vi "EnFlo_Seeder_Control.vi"(0 "Current Time (s)":dbl) -> ()   [LabVIEW 2014]
panel:
  in  "Minium Seeder power setting (Pmin)":dbl=27.0
  in  "Minimum Transducer Setting (Tmin)":dbl=6.0
  in  "Fluid Flowrate Factor":dbl=1.2 min=0.2 max=4.0 step=0.1 format="%.1g"
  in  "Sugar Strength":dbl=0.23
  out "Leak Detected or Emergency Stop":bool
  in  "Performing hand clean":bool
  out "Run Transducer":bool
  out "Sugar Pump":bool
  out "Low Flow":bool
  out "High Flow":bool
  out "Time Since Last Flush (min)":dbl
  out "Running Flush time":dbl
  out "Transducer setting":dbl
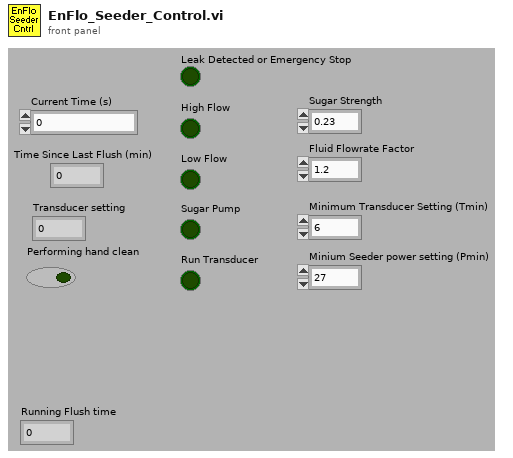
[diagram p1: front panel]
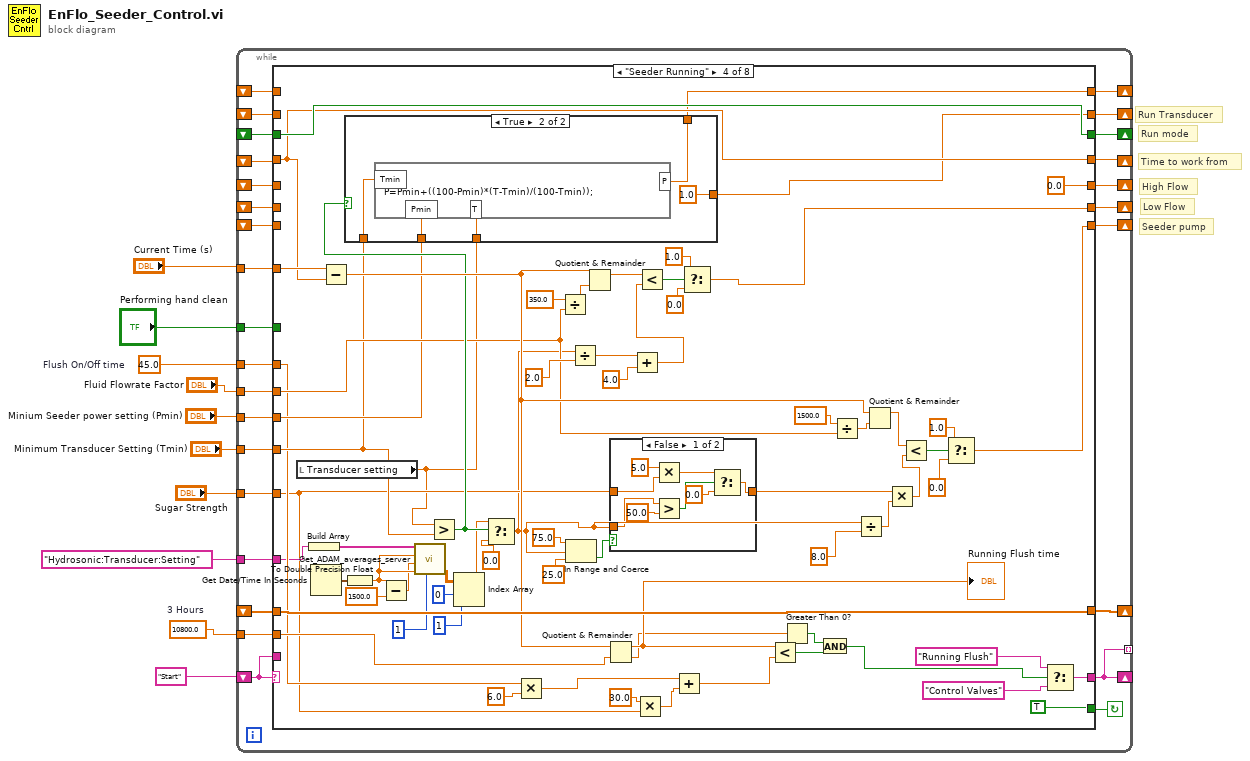
[diagram p0: block diagram]
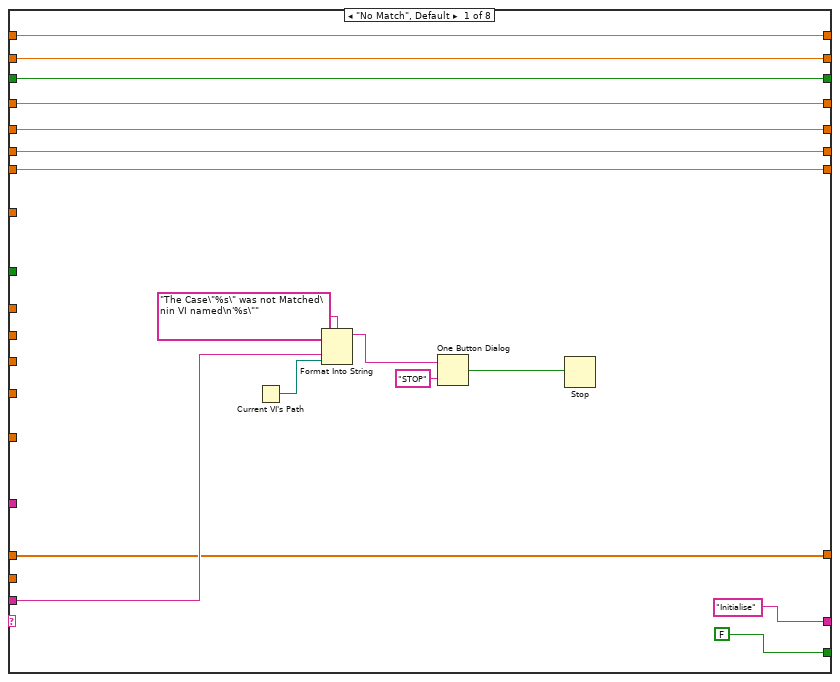
[diagram p2: hidden frame]
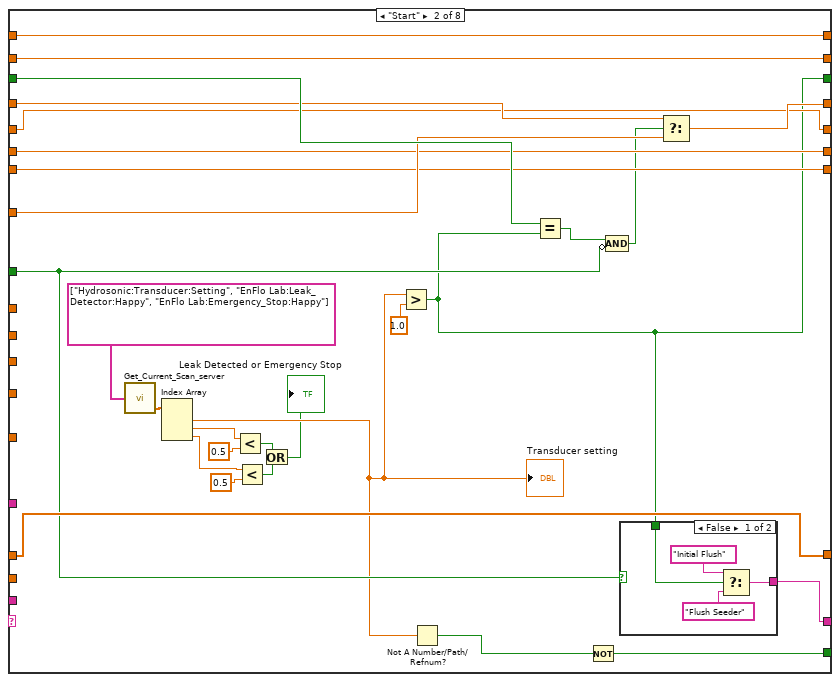
[diagram p3: hidden frame]
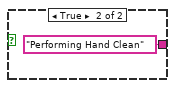
[diagram p4: hidden frame]
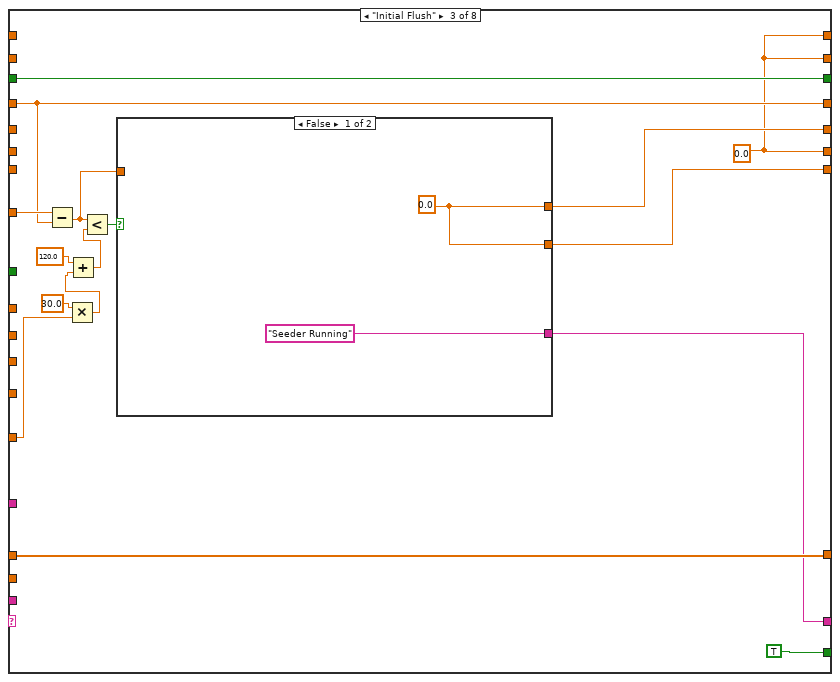
[diagram p5: hidden frame]
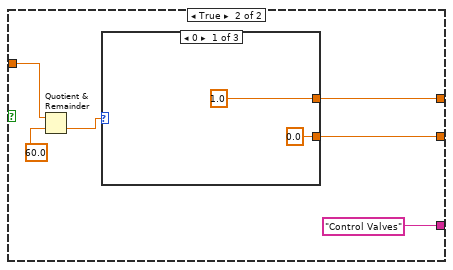
[diagram p6: hidden frame]
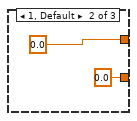
[diagram p7: hidden frame]
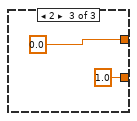
[diagram p8: hidden frame]
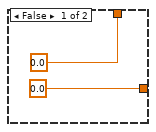
[diagram p10: hidden frame]
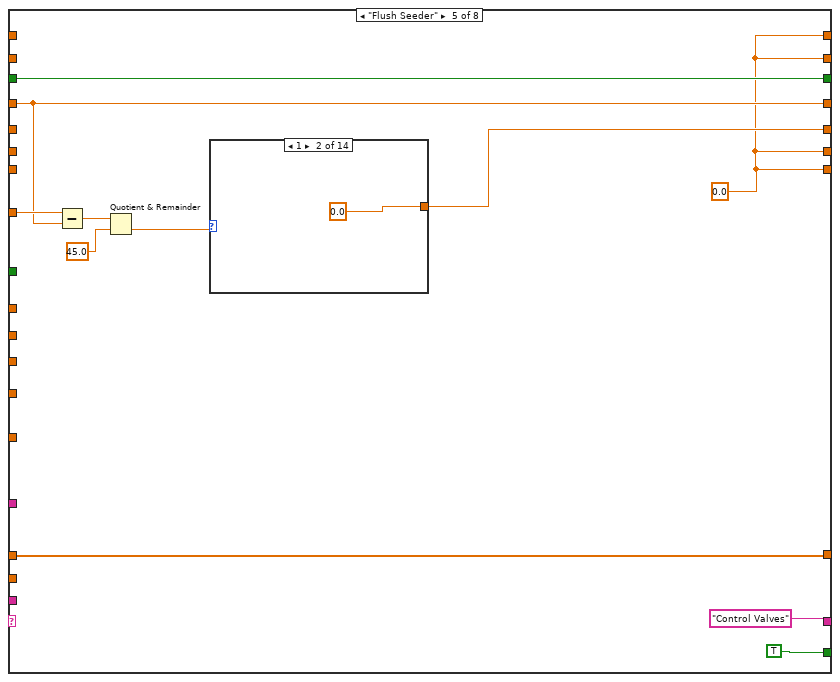
[diagram p11: hidden frame]
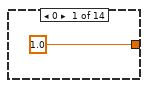
[diagram p12: hidden frame]
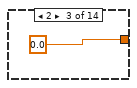
[diagram p13: hidden frame]
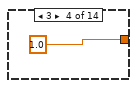
[diagram p14: hidden frame]
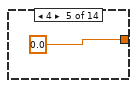
[diagram p15: hidden frame]
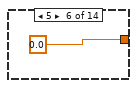
[diagram p16: hidden frame]
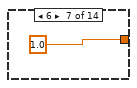
[diagram p17: hidden frame]
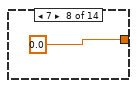
[diagram p18: hidden frame]
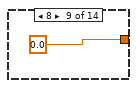
[diagram p19: hidden frame]
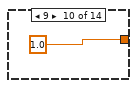
[diagram p20: hidden frame]
diagram:
  w2 = 45.0  # Flush On/Off time
  w8 = 10800.0  # 3 Hours
  # "Run Transducer"
  # "Seeder pump"
  # "Low Flow"
  # "High Flow"
  # "Run mode"
  # "Time to work from"
  n1 = while {
    shift-left: "Start" -> [w37]
    shift-right: [w21] -> _
    shift-right: [w36] -> _
    shift-left: _ -> [w33]
    shift-right: [w35] -> _
    shift-left: _ -> [w34]
    tunnel: "Current Time (s)" -> [w32]
    shift-right: [w30] -> _
    shift-left: _ -> [w31]
    shift-right: [w29] -> _
    shift-left: _ -> [w28]
    shift-right: [w26] -> _
    shift-left: _ -> [w27]
    shift-right: [w24] -> _
    shift-left: _ -> [w25]
    shift-right: [w23] -> _
    shift-left: _ -> [w22]
    tunnel: [w21] -> _ mode=indexing
    tunnel: w8 -> [w20]
    tunnel: "Performing hand clean" -> [w19]
    tunnel: "Sugar Strength" -> [w18]
    shift-right: [w17] -> _
    shift-left: _ -> [w16]
    tunnel: "Fluid Flowrate Factor" -> [w15]
    tunnel: "Minimum Transducer Setting (Tmin)" -> [w14]
    tunnel: "Minium Seeder power setting (Pmin)" -> [w13]
    tunnel: w2 -> [w12]
    tunnel: "Hydrosonic:Transducer:Setting" -> [w11]
    stop <- w38 continue-if-true
    n2 = case shown="\"Seeder Running\"" w37 {
      tunnel: [FALSE w80 TRUE TRUE TRUE TRUE TRUE FALSE] -> w38
      tunnel: ["Initialise" w75 w94 w164 "Control Valves" "Control Valves" "Control Valves" "End"] -> w21
      tunnel: w37 -> [w49 _ _ _ _ _ _ _]
      tunnel: [w44 w78 w97 w183 w208 w229 w243 w296] -> w36
      tunnel: [w46 w60 w102 w185 w210 w230 w244 w305] -> w35
      tunnel: w34 -> [w46 w79 w102 w185 w210 w230 w244 w305]
      tunnel: w33 -> [w44 w77 w97 w183 w208 w229 w243 w296]
      tunnel: w32 -> [_ w76 w98 w184 w209 _ _ w297]
      tunnel: w31 -> [w45 w74 _ _ _ _ _ w293]
      tunnel: [w45 w74 w101 0.0 w204 w227 w242 w293] -> w30
      tunnel: w28 -> [w43 w72 _ _ _ _ _ w291]
      tunnel: [w43 w72 w88 w173 w202 w227 w238 w291] -> w29
      tunnel: w27 -> [w42 w71 _ _ _ _ _ w289]
      tunnel: [w42 w71 w99 w167 w202 w227 w239 w289] -> w26
      tunnel: w25 -> [w41 w73 w100 w182 w203 w228 w241 w285]
      tunnel: [w41 w73 w100 w182 w203 w228 w241 w278] -> w24
      tunnel: w22 -> [w40 w70 _ _ _ _ _ w287]
      tunnel: [w40 w70 w88 w148 w202 w227 w238 w287] -> w23
      tunnel: w20 -> [_ _ _ w156 _ _ _ w281]
      tunnel: w19 -> [_ w67 _ _ _ _ _ _]
      tunnel: w18 -> [_ _ w91 w123 _ _ _ _]
      tunnel: [w39 w63 w88 w147 w202 w227 w238 w273] -> w17
      tunnel: w16 -> [w39 w63 _ _ _ _ _ w273]
      tunnel: w15 -> [_ _ _ w142 _ _ _ _]
      tunnel: w14 -> [_ _ _ w139 _ _ _ _]
      tunnel: w13 -> [_ _ _ w140 _ _ _ _]
      tunnel: w12 -> [_ _ _ w138 _ _ w237 _]
      tunnel: w11 -> [_ _ _ w135 _ _ _ _]
      frame "No Match", Default {
        n3 = Current VI's Path() -> (path=w48:path)
        n4 = Format Into String(format string="The Case\"%s\" was not Matched\nin VI named\n'%s\"" ("Format String"), w49, w48) -> (resulting string=w52:string)  [unwired: 2 in, 1 out]
        n5 = One Button Dialog(message=w52, button name ("OK")="STOP") -> (true=w50:bool)
        n6 = Stop(stop? (T)=w50) -> ()
      }
      frame "Start" {
        n7 = call "Get_Current_Scan_server.vi"("Desired Channels"=string[] ["Hydrosonic:Transducer:Setting", "EnFlo Lab:Leak_Detector:Happy", "EnFlo Lab:Emergency_Stop:Happy"] ("appended array")) -> ("Numerical Values"=w82:dbl[])  [unwired: 2 out]
        n8 = Index Array(array=w82) -> (element #1=w62:dbl, element #2=w65:dbl, element #3=w58:dbl)  [unwired: 3 in]
        "Transducer setting" <- w62
        n9 = Less?(x=w65, y=0.5) -> (x < y?=w56:bool)
        n10 = Less?(x=w58, y=0.5) -> (x < y?=w57:bool)
        n11 = Or(x=w56, y=w57) -> (x .or. y?=→"Leak Detected or Emergency Stop":bool)
        n12 = Greater?(x=w62, y=1.0) -> (0:w60:bool)
        n13 = Not A Number/Path/Refnum?(number/path/refnum=w62) -> (NaN/Path/Refnum?=w81:bool)
        n14 = Equal?(x=w79, y=w60) -> (x = y?=w69:bool)
        n15 = Not(x=w81) -> (.not. x?=w80:bool)
        n16 = Compound Arithmetic op=AND(w69, invert w67) -> (w68:bool)
        n17 = case shown="False" w67 {
          tunnel: w60 -> [w86 _]
          tunnel: [w85 "Performing Hand Clean"] -> w75
          frame False {
            n18 = Select(t="Initial Flush", s=w86, f="Flush Seeder") -> (s? t:f=w85:string)
          }
          frame True {
          }
        }
        n19 = Select(t=w77, s=w68, f=w76) -> (s? t:f=w78:dbl)
      }
      frame "Initial Flush" {
        w88 = 0.0
        n20 = Subtract(x=w98, y=w97) -> (x-y=w95:dbl)
        n21 = Multiply(x=30.0 ("y"), y=w91) -> (x*y=w90:dbl)
        n22 = Add(x=120.0 ("y"), y=w90) -> (x+y=w89:dbl)
        n23 = Less?(x=w95, y=w89) -> (x < y?=w96:bool)
        n24 = case shown="False" w96 {
          tunnel: [w105 w111] -> w101
          tunnel: [w105 w110] -> w99
          tunnel: w95 -> [_ w108]
          tunnel: ["Seeder Running" "Control Valves"] -> w94
          frame False {
            w105 = 0.0
          }
          frame True {
            n25 = Quotient & Remainder(x=w108, y=60.0) -> (floor(x/y)=w107:dbl)  [unwired: 1 out]
            n26 = case shown="0" w107 {
              tunnel: [1.0 0.0 0.0] -> w111
              tunnel: [0.0 0.0 1.0] -> w110
              frame 0 {
              }
              frame 1, Default {
              }
              frame 2 {
              }
            }
          }
        }
      }
      frame "Seeder Running" {
        n27 = local read "Transducer setting"() -> (w118:dbl)
        n28 = Build Array(w135) -> (w134:string[])
        n29 = Get Date/Time In Seconds() -> (seconds since 1Jan1904=w133:timestamp)
        n30 = Subtract(x=w184, y=w183) -> (x-y=w162:dbl)
        n31 = To Double Precision Float(number=w133) -> (double precision float=w132:dbl)
        n32 = Subtract(x=w132, y=1500.0) -> (x-y=w119:dbl)
        n33 = call "Get_ADAM_averages_server.vi"("No of averages"=1, "End time"=w132, "Start time"=w119, "Clients time"=w132, "ADAM Ch Names"=w134) -> ("DBL values"=w130:dbl[][])  [unwired: 1 in, 4 out]
        n34 = Greater?(x=w118, y=w139) -> (0:w149:bool)
        n35 = case shown="True" w149 {
          tunnel: [0.0 1.0] -> w148
          tunnel: [0.0 w198] -> w147
          tunnel: w140 -> [_ w200]
          tunnel: w139 -> [_ w199]
          tunnel: w118 -> [_ w197]
          frame False {
          }
          frame True {
            n36 = formula code="P=Pmin+((100-Pmin)*(T-Tmin)/(100-Tmin));"("Tmin"=w199, "T"=w197, "Pmin"=w200) -> ("P"=w198:dbl)
          }
        }
        n37 = Index Array(array=w130, index (row)=0, index (col)=1 ("disabled index (col)")) -> (element=w127:dbl)
        n38 = Select(t=w127, s=w149, f=0.0) -> (s? t:f=w121:dbl)
        n39 = Multiply(x=w138, y=6.0) -> (x*y=w136:dbl)
        n40 = Divide(x=350.0 ("y"), y=w142) -> (x/y=w144:dbl)
        n41 = In Range and Coerce(upper limit=75.0, x=w121, lower limit=25.0) -> (In Range?=w124:bool)  [unwired: 1 out]
        n42 = Divide(x=w121, y=2.0) -> (x/y=w146:dbl)
        n43 = Quotient & Remainder(x=w162, y=w144) -> (x-y*floor(x/y)=w181:dbl)  [unwired: 1 out]
        n44 = Quotient & Remainder(x=w162, y=w156) -> (x-y*floor(x/y)=w163:dbl, floor(x/y)=w160:dbl)
        "Running Flush time" <- w163
        n45 = case shown="False" w124 {
          tunnel: w123 -> [w187 w194]
          tunnel: [w191 w194] -> w122
          tunnel: w121 -> [w193 _]
          frame False {
            n46 = Multiply(x=5.0, y=w187) -> (x*y=w188:dbl)
            n47 = Greater?(x=w193, y=50.0) -> (0:w190:bool)
            n48 = Select(t=w188, s=w190, f=0.0) -> (s? t:f=w191:dbl)
          }
          frame True {
          }
        }
        n49 = Add(x=w146, y=4.0) -> (x+y=w176:dbl)
        n50 = Multiply(x=30.0 ("y"), y=w123) -> (x*y=w152:dbl)
        n51 = Less?(x=w181, y=w176) -> (x < y?=w180:bool)
        n52 = Add(x=w136, y=w152) -> (x+y=w151:dbl)
        n53 = Select(t=1.0, s=w180, f=0.0) -> (s? t:f=w173:dbl)
        n54 = Less?(x=w163, y=w151) -> (x < y?=w158:bool)
        n55 = Greater Than 0?(x=w160) -> (x > 0?=w159:bool)
        n56 = And(x=w159, y=w158) -> (x .and. y?=w157:bool)
        n57 = Divide(x=1500.0 ("y"), y=w142) -> (x/y=w141:dbl)
        n58 = Divide(x=w121, y=8.0) -> (x/y=w154:dbl)
        n59 = Quotient & Remainder(x=w162, y=w141) -> (x-y*floor(x/y)=w168:dbl)  [unwired: 1 out]
        n60 = Multiply(x=w122, y=w154) -> (x*y=w155:dbl)
        n61 = Less?(x=w168, y=w155) -> (x < y?=w169:bool)
        n62 = Select(t=1.0, s=w169, f=0.0) -> (s? t:f=w167:dbl)
        n63 = Select(t="Running Flush", s=w157, f="Control Valves") -> (s? t:f=w164:string)
      }
      frame "Flush Seeder" {
        w202 = 0.0
        n64 = Subtract(x=w209, y=w208) -> (x-y=w207:dbl)
        n65 = Quotient & Remainder(x=w207, y=45.0) -> (floor(x/y)=w205:dbl)  [unwired: 1 out]
        n66 = case shown="1" w205 {
          tunnel: [1.0 0.0 0.0 1.0 0.0 0.0 1.0 0.0 0.0 1.0 0.0 0.0 1.0 0.0] -> w204
          frame 0 {
          }
          frame 1 {
          }
          frame 2 {
          }
          frame 3 {
          }
          frame 4 {
          }
          frame 5 {
          }
          frame 6 {
          }
          frame 7 {
          }
          frame 8 {
          }
          frame 9 {
          }
          frame 10 {
          }
          frame 11 {
          }
          frame 12 {
          }
          frame 13, Default {
          }
        }
      }
      frame "Performing Hand Clean" {
        w227 = 0.0
      }
      frame "Running Flush" {
        w238 = 0.0
        n67 = local read "Running Flush time"() -> (w240:dbl)
        n68 = Quotient & Remainder(x=w240, y=w237) -> (floor(x/y)=w236:dbl)  [unwired: 1 out]
        n69 = To Long Integer(number=w236) -> (32bit integer=w233:i32)
        n70 = feedback-in #1(w233) -> ()
        n71 = feedback #1() -> (w235:i32)  [unwired: 1 in]
        n72 = Not Equal?(x=w233, y=w235) -> (x != y?=w234:bool)
        n73 = case shown="0" w233 {
          tunnel: [1.0 0.0 1.0 0.0 1.0 0.0 0.0] -> w242
          tunnel: [0.0 0.0 0.0 0.0 0.0 0.0 1.0] -> w239
          tunnel: w234 -> [_ _ _ _ _ _ w259]
          frame 0 {
          }
          frame 1 {
          }
          frame 2 {
          }
          frame 3 {
          }
          frame 4 {
          }
          frame 5, Default {
          }
          frame 6 {
            n74 = local read "Transducer setting"() -> (w262:dbl)
            n75 = In Range and Coerce(upper limit=90.0, x=w262, lower limit=8.0) -> (In Range?=w260:bool)  [unwired: 1 out]
            n76 = And(x=w260, y=w259) -> (x .and. y?=w261:bool)
            n77 = case shown="True" w261 {
              tunnel: w262 -> [_ w270]
              frame False {
              }
              frame True {
                n78 = Add(x=w270, y=10.0) -> (x+y=w267:dbl)
                n79 = Build Array("Hydrosonic:Transducer:Setting") -> (w271:string[])
                n80 = Build Array(w267) -> (w268:dbl[])
                n81 = call "ASYNC_Adam_server.vi"("Values"=w268, "Channel Names"=w271) -> ()  [unwired: 1 in, 3 out]
              }
            }
          }
        }
      }
      frame "Control Valves" {
        n82 = Subtract(x=w297, y=w296) -> (x-y=w282:dbl)
        n83 = local read "Leak Detected or Emergency Stop"() -> (w279:bool)
        n84 = Quotient & Remainder(x=w282, y=w281) -> (x-y*floor(x/y)=w280:dbl)  [unwired: 1 out]
        n85 = Divide(x=w280, y=60.0) -> (x/y=→"Time Since Last Flush (min)":dbl)
        n86 = Build Array(w287, w293, w291, w289, w273) -> (w275:dbl[])
        n87 = Array Size(array=w285) -> (size(s)=w284:i32)
        n88 = Equal To 0?(x=w284) -> (x = 0?=w283:bool)
        n89 = Array Size(array=w275) -> (size(s)=w277:i32)
        n90 = Initialize Array(0.0 ("element"), w277) -> (w274:dbl[])
        n91 = Select(t=w274, s=w279, f=w275) -> (s? t:f=w278:dbl[])
        n92 = case shown="False" w283 {
          tunnel: w278 -> [w310 w315]
          tunnel: string[] ["Hydrosonic:Seeder:Enable", "EnFlo_Tunnel:Seeder:High_Flow", "EnFlo_Tunnel:Seeder:Low_Flow", "EnFlo_Tunnel:Seeder_Pump:Enable", "EnFlo_Tunnel:Seeder:Power"] ("Desired Ch Names") -> [w309 w316]
          tunnel: [w308 w316] -> w301
          tunnel: [w307 w315] -> w300
          tunnel: w285 -> [w306 _]
          frame False {
            n93 = for {
              tunnel: w306 -> [w314] mode=indexing
              tunnel: w310 -> [w313] mode=indexing
              tunnel: [w313] -> w307 mode=indexing if=w311
              tunnel: w309 -> [w312] mode=indexing
              tunnel: [w312] -> w308 mode=indexing if=w311
              n94 = Not Equal?(x=w313, y=w314) -> (x != y?=w311:bool)
            }
          }
          frame True {
          }
        }
        n95 = Array Size(array=w300) -> (size(s)=w304:i32)
        n96 = Greater Than 0?(x=w304) -> (x > 0?=w303:bool)
        n97 = case shown="True" w303 {
          tunnel: w300 -> [_ w318]
          tunnel: w301 -> [_ w317]
          frame False {
          }
          frame True {
            n98 = call "ASYNC_Adam_server.vi"("Values"=w318, "Channel Names"=w317) -> ()  [unwired: 1 in, 3 out]
          }
        }
        n99 = Greater Than 0?(x=w293) -> (x > 0?=→"High Flow":bool)
        n100 = Greater Than 0?(x=w291) -> (x > 0?=→"Low Flow":bool)
        n101 = Greater Than 0?(x=w287) -> (x > 0?=→"Run Transducer":bool)
        n102 = Greater Than 0?(x=w289) -> (x > 0?=→"Sugar Pump":bool)
      }
    }
  }
